vi "DTM Read.vi"(7 "error in (no error)":errorcluster, 9 "Center ratio":dbl=1.0, 10 "VISA resource name":refnum<visa-resource-name>="GPIB0::2::INSTR") -> (0 "error out":errorcluster, 1 "Center Field":dbl format="%_2g", 2 "Read Field":dbl format="%_2g", 3 "read buffer":string)   [LabVIEW 2015]
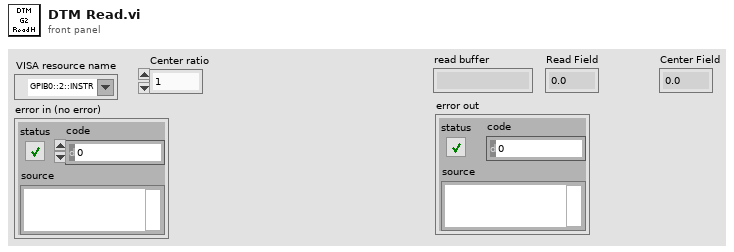
[diagram p1: front panel]
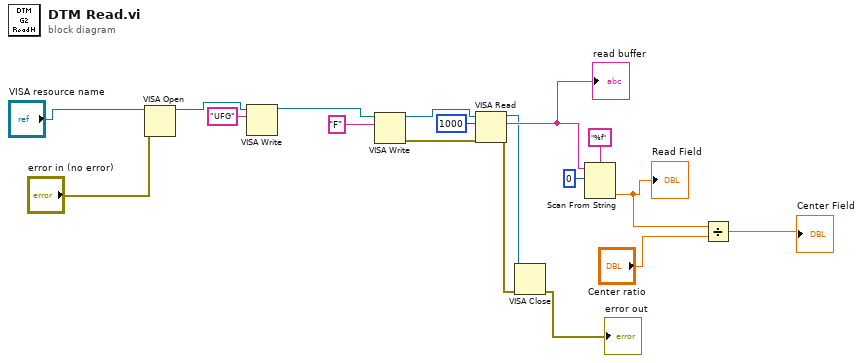
[diagram p0: block diagram]
diagram:
  n1 = VISA Open(error in (no error)="error in (no error)", VISA resource name="VISA resource name") -> (VISA resource name=w4:refnum<visa-resource-name>)  [unwired: 3 in, 1 out]
  n2 = VISA Write(VISA resource name=w4, write buffer="UFG") -> (VISA resource name out=w13:refnum<visa-resource-name>)  [unwired: 1 in, 2 out]
  n3 = VISA Write(VISA resource name=w13, write buffer="F") -> (VISA resource name out=w15:refnum<visa-resource-name>, error out=w14:errorcluster)  [unwired: 1 in, 1 out]
  n4 = VISA Read(VISA resource name=w15, byte count=u32 1000, error in (no error)=w14) -> (VISA resource name out=w8:refnum<visa-resource-name>, read buffer=w10:string, error out=w7:errorcluster)  [unwired: 1 out]
  "read buffer" <- w10
  n5 = VISA Close(VISA resource name=w8, error in (no error)=w7) -> (error out=→"error out":errorcluster)
  n6 = Scan From String(format string="%f", input string=w10, initial scan location=u32 0) -> (output 1=w3:dbl)  [unwired: 2 in, 3 out]
  "Read Field" <- w3
  n7 = Divide(x=w3, y="Center ratio") -> (x/y=→"Center Field":dbl)
